vi "ReadSizeMat_2DArray-I32.vi"(8 "error in":errorcluster, 11 "Array in":i16[][](array[numeric])) -> (0 "error out":errorcluster, 1 "Height":i32, 2 "Width":i32, 3 "Array out":i16[][](array[numeric]), 4 "Channel":i32)   [LabVIEW 2020, in "OpenLvVision_OpenCv.lvlib"]
doc: "Read size of the datatype\nNo malleable to breake vi inlining!"
uses:
  OpenLvVision_OpenCv.lvlib
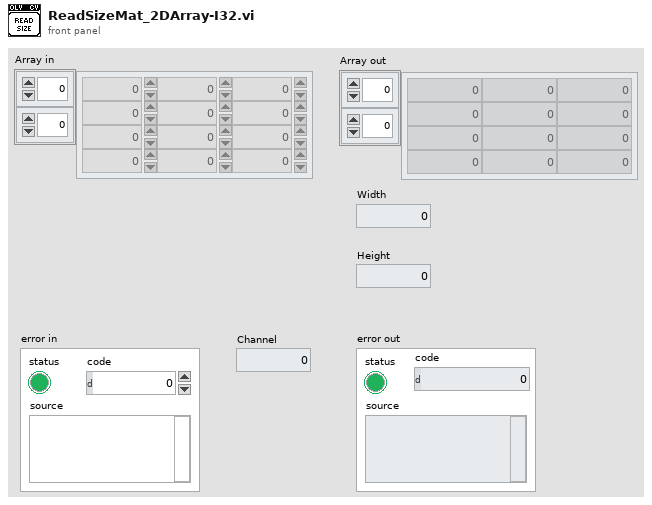
[diagram p1: front panel]
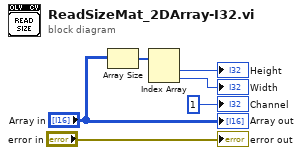
[diagram p0: block diagram]
diagram:
  n1 = Array Size(array="Array in") -> (size(s)=w4:i32[])
  n2 = Index Array(array=w4) -> (element #1=→"Height":i32, element #2=→"Width":i32)  [unwired: 2 in]
  "error out" <- "error in"
  "Channel" <- 1 ("Channel")
  "Array out" <- "Array in"
